vi "EditOptions.vi"(8 "error in":errorcluster, 11 "node in":refnum<class "Page.lvclass">) -> (0 "error out":errorcluster, 1 "edit options":T1, 2 "subnodes class":T2, 3 "node out":refnum<class "Page.lvclass">)   [LabVIEW 2019, in "Page.lvclass"]
doc: "Contains the options for the Menu that will be displayed when doing right click on an item.\nThe sub nodes class configures which nodes can be added to this nodes\nAnd the edit options determine which options are available for the node.\nThis configuration is stored in this VI in case some dynamic configuration is required for the menu options or sub nodes."
uses:
  Page.lvclass
  C:/Program Files (x86)/National Instruments/LabVIEW 2019/vi.lib/NI/Configuration Framework/Node/NISE_CEF_Node.lvclass
  <vilib>/NI/Configuration Framework/Node/SubNodeCluster.ctl
  <vilib>/NI/Configuration Framework/Node/NodeMenuOptions.ctl
  <vilib>/NI/Configuration Framework/Node/NISE_CEF_Node.lvclass/NISE_CEF_Node.ctl
  RunTimeObjects/RunTimeObjectsSection.lvclass
  RunTimeObjects/RunTimeObjectsSection.lvclass/RunTimeObjectsSection.ctl
  RunTimeObjects/Read RunTimeObjectType.vi
  <vilib>/NI/Configuration Framework/Node/ReadChildren.vi
  <vilib>/NI/Configuration Framework/Node/NISE_CEF_Node.lvclass
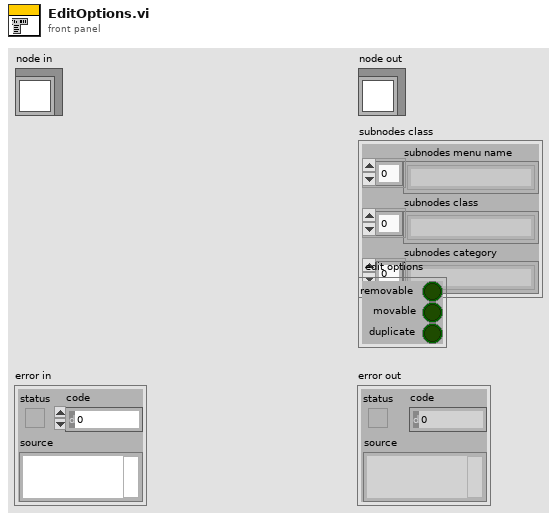
[diagram p1: front panel]
types:
  T1 = typedef "NISE_CEF_Node.lvclass/NodeMenuOptions.ctl" = cluster{"removable":bool, "movable":bool, "duplicate":bool}
  T2 = typedef "NISE_CEF_Node.lvclass/SubNodeCluster.ctl" = cluster{"subnodes menu name":string[], "subnodes class":string[], "subnodes category":string[]}
  T3 = typedef "NISE_CEF_Node.lvclass/NodeRef.ctl" = refnum<data-value>
  T4 = typedef "Configuration Tool.lvlib/RunTimeObjectTypes.ctl" = enum16{"ActionVIs", "ButtonList", "RunTimeMenu"}
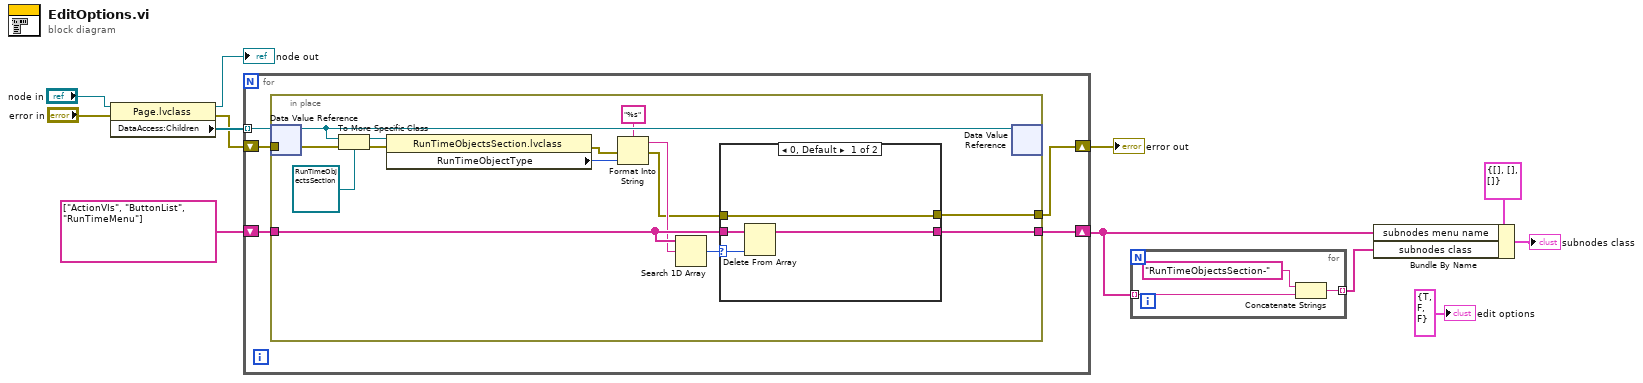
[diagram p0: block diagram]
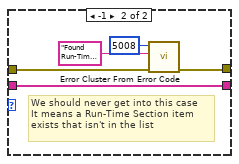
[diagram p2: hidden frame]
diagram:
  n1 = property class="Page.lvclass"(reference="node in", error in="error in") -> (reference out=→"node out":refnum<class "Page.lvclass">, error out=w7:errorcluster, "DataAccess:Children"=w8:T3[])
  n2 = for {
    tunnel: w8 -> [w17] mode=indexing
    shift-right: [w13] -> w3
    shift-left: w7 -> [w16]
    shift-right: [w14] -> w2
    shift-left: string[] ["ActionVIs", "ButtonList", "RunTimeMenu"] -> [w15]
    n3 = in-place {
      in-place-border: w16 -> [w30]
      in-place-border: w15 -> [w22]
      in-place-border: [w19] -> w14
      in-place-border: [w18] -> w13
      n4 = in-place-dvr #1(w17) -> (w31:refnum<class "NISE_CEF_Node.lvclass">)  [unwired: 1 out]
      n5 = To More Specific Class(target class=refnum<class "RunTimeObjectsSection.lvclass"> refnum ("RunTimeObjectsSection.lvclass"), reference=w31, error in=w30) -> (specific class reference=w28:refnum<class "RunTimeObjectsSection.lvclass">, error out=w27:errorcluster)
      n6 = property class="RunTimeObjectsSection.lvclass"(reference=w28, error in=w27) -> (error out=w25:errorcluster, "RunTimeObjectType"=w26:T4)  [unwired: 1 out]
      n7 = Format Into String(format string="%s", error in=w25, w26) -> (resulting string=w21:string, error out=w20:errorcluster)  [unwired: 1 in]
      n8 = Search 1D Array(1D array=w22, element=w21) -> (index of element=w23:i32)  [unwired: 1 in]
      n9 = case shown="0, Default" w23 {
        selector: w23 -> [w33 _]
        tunnel: w22 -> [w35 w40]
        tunnel: [w34 w40] -> w19
        tunnel: w20 -> [w32 w39]
        tunnel: [w32 w36] -> w18
        frame 0, Default {
          n10 = Delete From Array(array=w35, index=w33) -> (array with subset deleted=w34:string[])  [unwired: 1 in, 1 out]
        }
        frame -1 {
          # "We should never get into this case\nIt means a Run-Time Section item \nexists that isn't in the list"
          n11 = call <vilib>:"Error Cluster From Error Code.vi"("error in (no error)"=w39, "error message (\"\")"="Found Run-Time Section Object we weren't expecting" ("error message (\"\")"), "error code (0)"=5008) -> ("error out"=w36:errorcluster)  [unwired: 6 in]
        }
      }
      n12 = in-place-dvr #1(w31) -> ()  [unwired: 2 out]
    }
  }
  "error out" <- w3
  n13 = for {
    tunnel: w2 -> [w42] mode=indexing
    tunnel: [w41] -> w1 mode=indexing
    n14 = Concatenate Strings("RunTimeObjectsSection-", w42) -> (w41:string)
  }
  n15 = Bundle By Name(cluster=T2 {"subnodes menu name"=[], "subnodes class"=[], "subnodes category"=[]} ("subnodes class"), "subnodes menu name"=w2, "subnodes class"=w1) -> (→"subnodes class":T2)
  "edit options" <- T1 {"removable"=TRUE, "movable"=FALSE, "duplicate"=FALSE} ("edit options")
